vi "SetGridParam (SubVI).vi"(8 "error in (no error)":errorcluster, 10 "GridSettings":T2, 11 "Application in":refnum<vi>) -> (0 "Error out":errorcluster, 3 "Application ref out":refnum<vi>)   [LabVIEW 2014]
uses:
  <userlib>/Nanonis Prog Interface V5/Scan/Grid/GridPatternGet.vi
  <userlib>/Nanonis Prog Interface V5/Scan/Grid/GridPatternSet.vi
  <userlib>/Nanonis Prog Interface V5/Nanonis Prog Interface.lvlib
panel:
  in  "Multiple sweeps config":T1
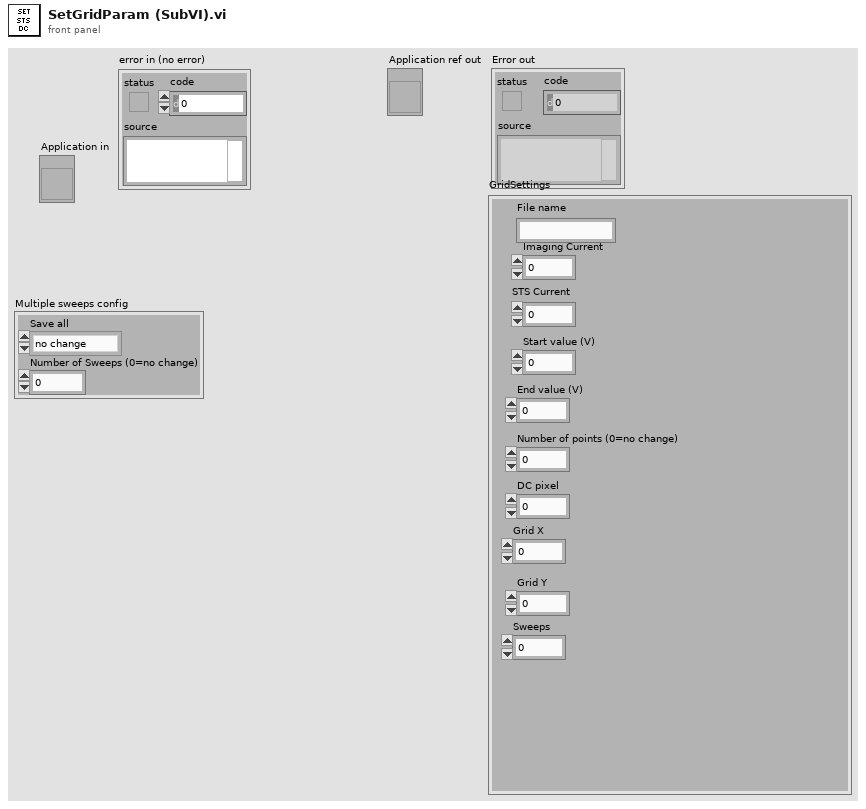
[diagram p1: front panel]
types:
  T1 = cluster{"Save all":enum16{"no change", "on", "off"}, "Number of Sweeps (0=no change)":i32}
  T2 = cluster{"Imaging Current":sgl, "STS Current":sgl, "Start value (V)":sgl, "End value (V)":sgl, "Number of points (0=no change)":i32, "File name":string, "DC pixel":dbl, "Grid X":dbl, "Grid Y":dbl, "Sweeps":dbl}
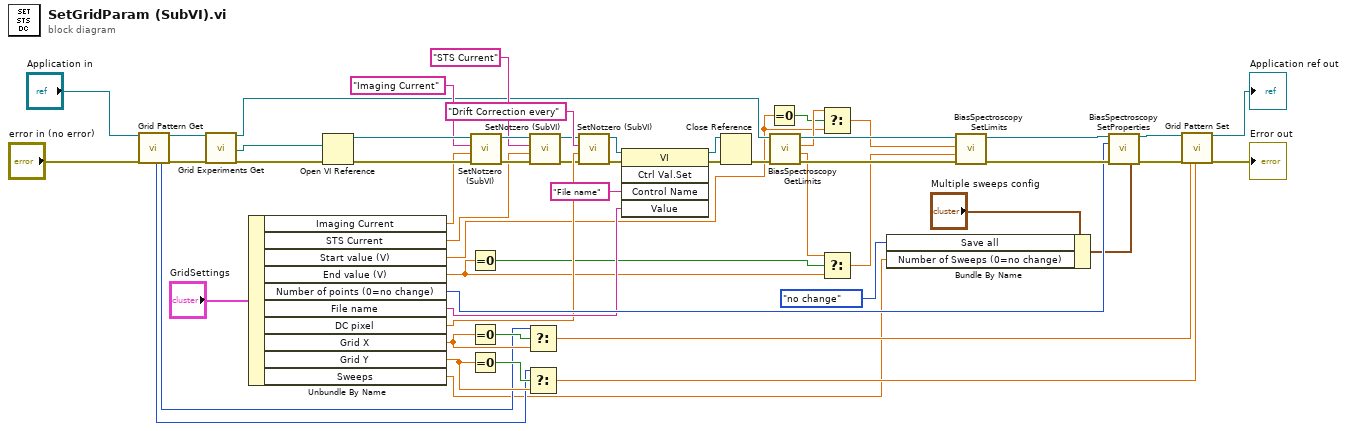
[diagram p0: block diagram]
diagram:
  n1 = call-poly <userlib>:"Grid Pattern Get.vi"("Application ref in"="Application in", "error in (no error)"="error in (no error)") -> ("Points Y"=w32:i32, "Points X"=w31:i32, "Application ref out"=w37:refnum<vi>, "error out"=w39:errorcluster)  [unwired: 9 in, 5 out]
  n2 = call <userlib>:"Grid Experiments Get.vi"("Application ref in"=w37, "error in (no error)"=w39) -> ("Application ref out"=w12:refnum<vi>, "External VI path"=w54:path, "error out"=w51:errorcluster)  [unwired: 11 in, 4 out]
  n3 = Unbundle By Name("GridSettings") -> ("Imaging Current"=w23:sgl, "STS Current"=w13:sgl, "Start value (V)"=w2:sgl, "End value (V)"=w1:sgl, "Number of points (0=no change)"=w49:i32, "File name"=w45:string, "DC pixel"=w19:dbl, "Grid X"=w34:dbl, "Grid Y"=w33:dbl, "Sweeps"=w26:dbl)
  n4 = Open VI Reference(vi path=w54, error in (no error)=w51) -> (vi reference=w55:refnum<vi>, error out=w52:errorcluster)  [unwired: 4 in]
  n5 = Equal To 0?(x=w1) -> (x = 0?=w4:bool)
  n6 = Equal To 0?(x=w34) -> (x = 0?=w36:bool)
  n7 = Equal To 0?(x=w33) -> (x = 0?=w35:bool)
  n8 = call "SetNotzero (SubVI).vi"("error in (no error)"=w52, "Value"=w23, "Control Name"="Imaging Current", "VI in"=w55) -> ("error out"=w15:errorcluster, "VI out"=w18:refnum<vi>)  [unwired: 6 in]
  n9 = Select(t=w31, s=w36, f=w34) -> (s? t:f=w29:dbl)
  n10 = Select(t=w32, s=w35, f=w33) -> (s? t:f=w30:dbl)
  n11 = call "SetNotzero (SubVI).vi"("error in (no error)"=w15, "Value"=w13, "Control Name"="STS Current", "VI in"=w18) -> ("error out"=w16:errorcluster, "VI out"=w17:refnum<vi>)  [unwired: 6 in]
  n12 = call "SetNotzero (SubVI).vi"("error in (no error)"=w16, "Value"=w19, "Control Name"="Drift Correction every", "VI in"=w17) -> ("error out"=w21:errorcluster, "VI out"=w22:refnum<vi>)  [unwired: 6 in]
  n13 = invoke class="VI" method="Ctrl Val.Set"(reference=w22, error in=w21, "Control Name"="File name", "Value"=w45) -> (reference out=w47:refnum<vi>, error out=w48:errorcluster)  [unwired: 1 in, 3 out]
  n14 = Close Reference(reference=w47, error in (no error)=w48) -> (error out=w11:errorcluster)
  n15 = Equal To 0?(x=w2) -> (x = 0?=w3:bool)
  n16 = call <userlib>:"BiasSpectroscopy GetLimits.vi"("Error in (no error)"=w11, "Application ref in"=w12) -> ("Error out"=w10:errorcluster, "End value (V)"=w7:sgl, "Start value (V)"=w8:sgl, "Application ref out"=w9:refnum<vi>)  [unwired: 4 in]
  n17 = Select(t=w8, s=w3, f=w2) -> (s? t:f=w5:sgl)
  n18 = Select(t=w7, s=w4, f=w1) -> (s? t:f=w6:sgl)
  n19 = Bundle By Name(cluster="Multiple sweeps config", "Save all"=enum16{"no change", "on", "off"}."no change", "Number of Sweeps (0=no change)"=w26) -> (w25:T1)
  n20 = call <userlib>:"BiasSpectroscopy SetLimits.vi"("Error in (no error)"=w10, "End value (V)"=w6, "Start value (V)"=w5, "Application ref in"=w9) -> ("Error out"=w53:errorcluster, "Application ref out"=w56:refnum<vi>)  [unwired: 4 in]
  n21 = call <userlib>:"BiasSpectroscopy SetProperties.vi"("Application ref in"=w56, "Number of points (0=no change)"=w49, "Error in (no error)"=w53, "Multiple sweeps config"=w25) -> ("Application ref out"=w44:refnum<vi>, "Error out"=w42:errorcluster)  [unwired: 10 in]
  n22 = call-poly <userlib>:"Grid Pattern Set.vi"("Application ref in"=w44, "error in (no error)"=w42, "Points X"=w29, "Points Y"=w30) -> ("Application ref out"=→"Application ref out":refnum<vi>, "error out"=→"Error out":errorcluster)  [unwired: 14 in]
